vi "Search Device wrapper.vi"(8 "error in (no error)":errorcluster caption="错误输入（无错误）", 10 "pGWSearchPara":cluster{"dwComIndex":u32, "dwBtr":u32}, 11 "dwDevType":u32(ring)=4 items=["USBCAN"=4, "WIFI2RS232CAN"=2, "RS232CAN"=1]) -> (0 "error out":errorcluster caption="错误输出", 2 "pGWSearchPara out":cluster{"dwComIndex":u32, "dwBtr":u32}, 3 "function return":u32)   [LabVIEW 2016, in "UISimCanFunc_wrapper.lvlib"]
doc: "_declspec (dllexport) DWORD SearchDevice_wrapper(DWORD dwDevType, P_GW_SEARCH_PARA pGWSearchPara);"
uses:
  <userlib>/UISimCanFunc_wrapper/UISimCanFunc_wrapper.lvlib
  <userlib>/UISimCanFunc_wrapper/UISimCanFunc_wrapper.dll
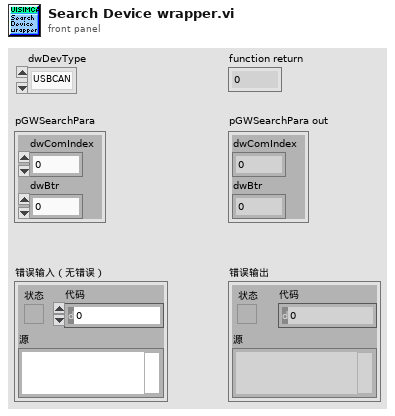
[diagram p1: front panel]
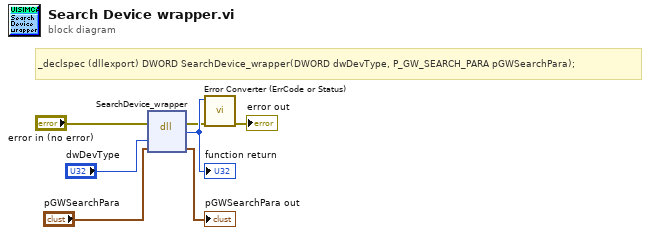
[diagram p0: block diagram]
diagram:
  # "_declspec (dllexport) DWORD SearchDevice_wrapper(DWORD dwDevType, P_GW_SEARCH_PARA pGWSearchPara);"
  n1 = dll-call lib="C:/Program Files (x86)/National Instruments/LabVIEW 2016/user.lib/UISimCanFunc_wrapper/UISimCanFunc_wrapper.*" fn="SearchDevice_wrapper"(error in="error in (no error)", "dwDevType"="dwDevType", "pGWSearchPara"="pGWSearchPara") -> (error out=w2:errorcluster, w7:u32, "pGWSearchPara"=→"pGWSearchPara out":cluster{"dwComIndex":u32, "dwBtr":u32})  [unwired: 3 in, 1 out]
  "function return" <- w7
  n2 = call <userlib>:"Error Converter (ErrCode or Status).vi"("error in (no error)"=w2, "error code"=w7) -> ("error out"=→"error out":errorcluster)  [unwired: 9 in]
